vi "TL behavior S-WallUPDATE.vi"(1 "Behavior\nVelocity":dbl, 2 "Activate?":bool=TRUE, 3 "Sensor":T1) -> (0 "S-Wall Array":dbl[](array[numeric]))   [LabVIEW 2014]
uses:
  sensorsSTD.ctl
  <vilib>/addons/control/pid/pid.llb/PID (DBL).vi
  <vilib>/addons/control/pid/NI_PID_pid.lvlib
panel:
  in  "setpoint 90deg":dbl=30.0 format="%#_13g"
  out "steer 90":dbl format="%.2f"
  out "Sensor B":string
  out "Sensor A":string
  in  "setpoint 45deg":dbl=45.0 format="%#_13g"
  out "steer 45":dbl format="%.2f"
  out "Waveform Graph":cluster{dbl, dbl, dbl[]}(graph)
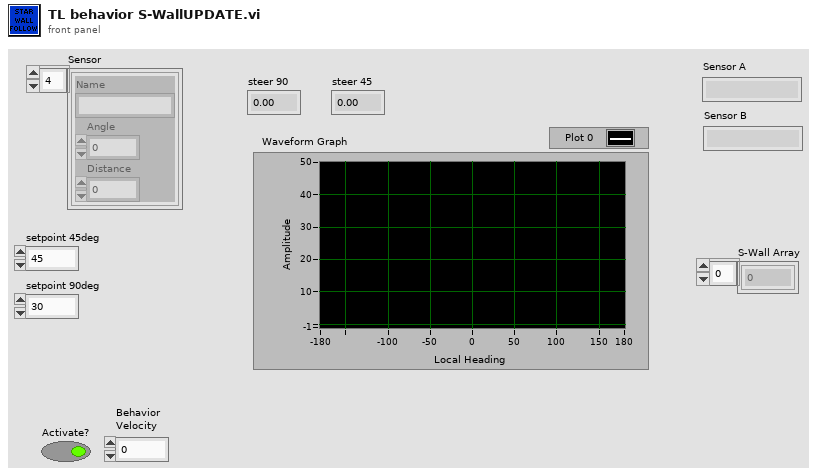
[diagram p1: front panel]
types:
  T1 = typedef "sensorsSTD.ctl" = cluster{"Name":string, "Angle":dbl, "Distance":dbl}[]
  T2 = cluster{"proportional gain (Kc)":dbl, "integral time (Ti, min)":dbl, "derivative time (Td, min)":dbl}
  T3 = cluster{"Name":string, "Angle":dbl, "Distance":dbl}
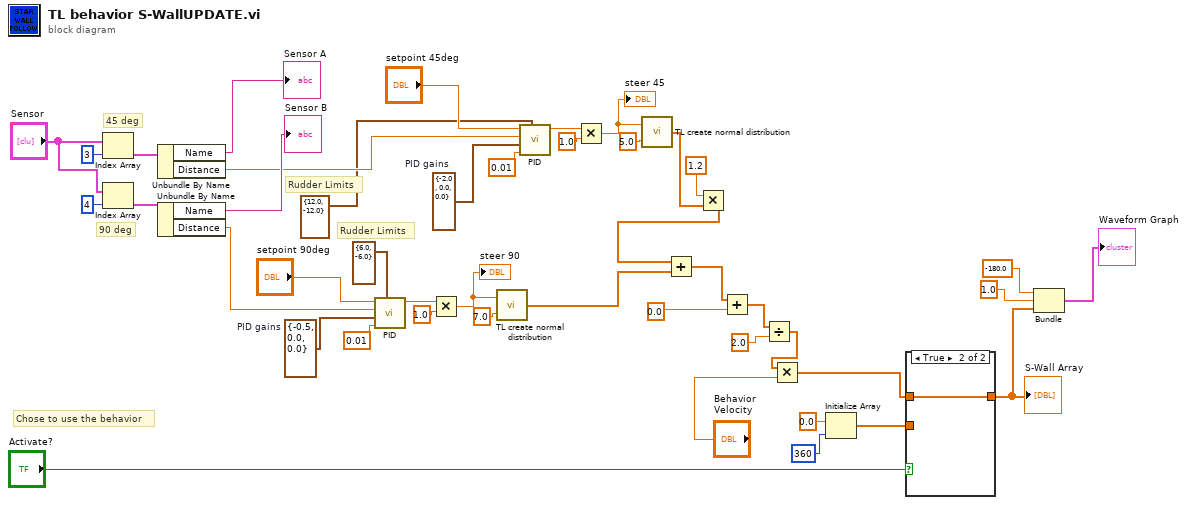
[diagram p0: block diagram]
diagram:
  w21 = T2 {"proportional gain (Kc)"=-0.5, "integral time (Ti, min)"=0.0, "derivative time (Td, min)"=0.0}  # PID gains
  w29 = T2 {"proportional gain (Kc)"=-2.0, "integral time (Ti, min)"=0.0, "derivative time (Td, min)"=0.0}  # PID gains
  # "Rudder Limits"
  # "90 deg"
  # "45 deg"
  # "Rudder Limits"
  # "Chose to use the behavior"
  n1 = Index Array(array="Sensor", index=3) -> (element=w43:T3)
  n2 = Index Array(array="Sensor", index=4) -> (element=w33:T3)
  n3 = Unbundle By Name(w43) -> ("Name"=→"Sensor A":string, "Distance"=w17:dbl)
  n4 = Unbundle By Name(w33) -> ("Name"=→"Sensor B":string, "Distance"=w18:dbl)
  n5 = call-poly <vilib>:"PID.vi"("output range"=cluster{"output high":dbl, "output low":dbl} {"output high"=6.0, "output low"=-6.0}, "dt (s)"=0.01, "PID gains"=w21, "process variable"=w18, "setpoint"="setpoint 90deg") -> ("output"=w24:dbl)  [unwired: 5 in, 1 out]
  n6 = Multiply(x=w24, y=1.0) -> (x*y=w20:dbl)
  "steer 90" <- w20
  n7 = call "TL create normal distribution.vi"("std (Normal)"=7.0, "mean"=w20) -> ("ACT array"=w15:dbl[])
  n8 = call-poly <vilib>:"PID.vi"("output range"=cluster{"output high":dbl, "output low":dbl} {"output high"=12.0, "output low"=-12.0}, "dt (s)"=0.01, "PID gains"=w29, "process variable"=w17, "setpoint"="setpoint 45deg") -> ("output"=w32:dbl)  [unwired: 5 in, 1 out]
  n9 = Multiply(x=w32, y=1.0) -> (x*y=w28:dbl)
  "steer 45" <- w28
  n10 = call "TL create normal distribution.vi"("std (Normal)"=5.0, "mean"=w28) -> ("ACT array"=w16:dbl[])
  n11 = Multiply(x=1.2, y=w16) -> (x*y=w2:dbl[])
  n12 = Add(x=w2, y=w15) -> (x+y=w9:dbl[])
  n13 = Add(x=w9, y=0.0) -> (x+y=w7:dbl[])
  n14 = Divide(x=w7, y=2.0) -> (x/y=w6:dbl[])
  n15 = Multiply(x=w6, y="Behavior\nVelocity") -> (x*y=w13:dbl[])
  n16 = Initialize Array(0.0 ("element"), 360 ("dimension size")) -> (w36:dbl[])
  n17 = case shown="True" "Activate?" {
    tunnel: w36 -> [w45 _]
    tunnel: w13 -> [_ w46]
    tunnel: [w45 w46] -> w35
    frame False {
    }
    frame True {
    }
  }
  "S-Wall Array" <- w35
  n18 = Bundle(-180.0, 1.0, w35) -> (→"Waveform Graph":cluster{dbl, dbl, dbl[]})  [unwired: 1 in]
